vi "commit settings.vi"(8 "error in (no error)":errorcluster, 11 "PackedLibrary in":refnum<class "PackedLibrary.lvclass">) -> (0 "error out":errorcluster, 2 "Destinations":T1[](array[typedef]), 3 "Builder out":refnum<class "PackedLibrary.lvclass">)   [LabVIEW 2024, in "PackedLibrary.lvclass"]
uses:
  PackedLibrary.lvclass
  PackedLibrary.lvclass/PackedLibrary.ctl
  parent/Builder.lvclass
  <vilib>/AppBuilder/AB_API/PPL/NI_AB_API_PPL.lvclass
  <vilib>/AppBuilder/AB_API/common/AB_API Destination Type.ctl
  <vilib>/AppBuilder/AB_API/common/AB_API Destination Data.ctl
  D:/_repos/sandbox/github_p/labview-tools/cicd_tools/src/builders/parent/Builder.lvclass
  D:/_repos/sandbox/github_p/labview-tools/cicd_tools/src/builders/packed_library/PackedLibrary.lvclass
  C:/Program Files/National Instruments/LabVIEW 2024/vi.lib/AppBuilder/AB_API/Targetfile/NI_AB_API_Targetfile.lvclass
  C:/Program Files/National Instruments/LabVIEW 2024/vi.lib/AppBuilder/AB_API/Build/NI_AB_API_Build.lvclass
  C:/Program Files/National Instruments/LabVIEW 2024/vi.lib/AppBuilder/AB_API/PPL/NI_AB_API_PPL.lvclass
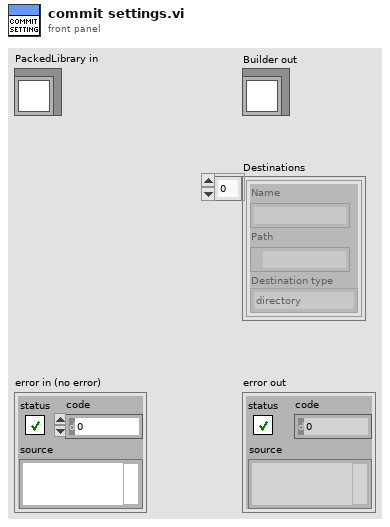
[diagram p1: front panel]
types:
  T1 = typedef "AB_API Destination Data.ctl" = cluster{"Name":string, "Path":path, "Destination type":T2}
  T2 = typedef "AB_API Destination Type.ctl" = enum16{"directory", "directory (preserve hierarchy)", "LLB"}
  T3 = typedef "AB_API Version Number.ctl" = cluster{"Major":u16, "Minor":u16, "Fix":u16, "Build":u16}
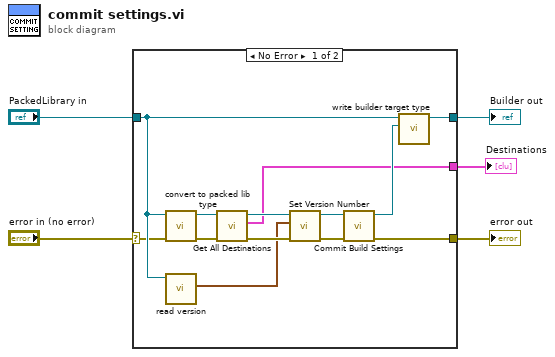
[diagram p0: block diagram]
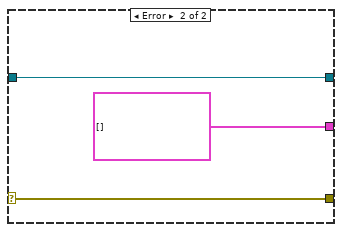
[diagram p2: hidden frame]
diagram:
  n1 = case shown="No Error" "error in (no error)" {
    selector: "error in (no error)" -> [w7 w21]
    tunnel: [w14 w21] -> w3
    tunnel: "PackedLibrary in" -> [w10 w20]
    tunnel: [w8 w20] -> w2
    tunnel: [w6 T1[] [] ("Destinations")] -> w1
    frame No Error {
      n2 = call "convert to packed lib type.vi"("error in (no error)"=w7, "PackedLibrary in"=w10) -> ("error out"=w12:errorcluster, "NI_AB_API_PPL out"=w11:refnum<class "NI_AB_API_PPL.lvclass">)  [unwired: 8 in]
      n3 = call "read version.vi"("Builder in"=w10) -> ("version"=w13:T3)  [unwired: 10 in]
      n4 = call-dynamic "Get All Destinations.vi"("error in (no error)"=w12, "NI_AB_API_Build in"=w11) -> ("error out"=w17:errorcluster, "Destinations"=w6:T1[], "NI_AB_API_Build out"=w18:refnum<class "NI_AB_API_PPL.lvclass">)  [unwired: 7 in]
      n5 = call-dynamic "Set Version Number.vi"("error in (no error)"=w17, "Version number"=w13, "PPL in"=w18) -> ("error out"=w15:errorcluster, "PPL out"=w16:refnum<class "NI_AB_API_PPL.lvclass">)  [unwired: 7 in]
      n6 = call-dynamic "Commit Build Settings.vi"("error in (no error)"=w15, "PPL in"=w16) -> ("error out"=w14:errorcluster, "PPL out"=w9:refnum<class "NI_AB_API_PPL.lvclass">)  [unwired: 8 in]
      n7 = call "write builder target type.vi"("builder target type"=w9, "Builder in"=w10) -> ("Builder out"=w8:refnum<class "PackedLibrary.lvclass">)  [unwired: 9 in]
    }
    frame Error {
    }
  }
  "error out" <- w3
  "Builder out" <- w2
  "Destinations" <- w1
